vi "LINX - PmodACL2.vi"() -> ()   [LabVIEW 2011]
doc: "PmodACL2\n\nThis example demonstrates how to read 3-axis acceleration values and temperature. \n\nInstructions:\n1. Select the COM Port associated with the LINX device\n2. Select the SPI Channel that the Pmod is connected to.\n3. Select the CS Channel that the Pmod is connected to.\n4. Use the controls to select resolution and data rate\n5. Click the Run Arrow."
uses:
  vi.lib/MakerHub/LINX/Public/Utilities/Open Serial.vi
  vi.lib/MakerHub/LINX/LMH-LINX.lvlib
  vi.lib/MakerHub/LINX/Public/Sensors/Pmods/ACL2/PmodACL2.lvlib
panel:
  out "Loop Rate (Hz)":u32
  out "Waveform Chart":T1(graph)
  in  "Stop Button":bool
  out "Temperature":dbl format="%#_3g"
  in  "Output Data Rate (Hz)":enum16{"400", "200", "100", "50", "25", "12.5"}(ring)=enum."100"
  in  "SPI Channel (0)":u8
  in  "Resolution (g)":enum16{"8g", "4g", "2g"}(ring)=enum."2g"
  in  "CS Channel":u8=10
  in  "Serial Port":refnum<visa-resource-name>="N/A"
  # "PmodACL2\n\nThis example demonstrates how to read 3-axis acceleration values and temperature from PmodACL2. \n\nInstructions:\n1. Select the COM Port associated with the LINX device\n2. Select the SPI Channel that the Pmod is connected to.\n3. Select the CS Channel that the Pmod is connected to.\n4. Use the controls to select resolution and data rate\n5. Click the Run Arrow."
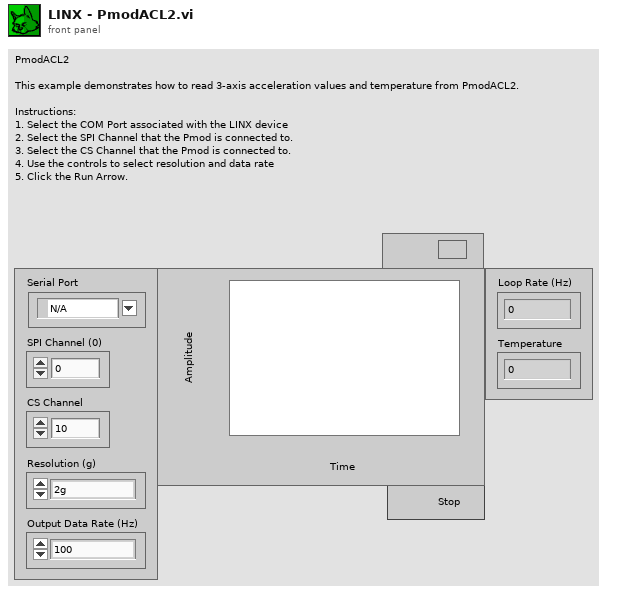
[diagram p1: front panel]
types:
  T1 = cluster{"Numeric Control":dbl, "Numeric Control":dbl, "Numeric Control":dbl}
  T2 = typedef "LMH-LINX.lvlib/LINX Ref.ctl" = cluster{"IO":T3, "Interface":T4, "LINX Device Config":T5}
  T3 = typedef "LMH-LINX.lvlib/Platform.ctl" = enum16{"Remote", "Local"}
  T4 = typedef "LMH-LINX.lvlib/Interface.ctl" = enum16{"Serial", "TCP"}
  T5 = typedef "LMH-LINX.lvlib/Device.lvlib/LINX Device Config.ctl" = cluster{"Interface":T4, "COM Port":refnum<visa-resource-name>, "TCP Configuration":T6, "Device Family":u8, "Device ID":u8, "Device Name":string, "TCP Ref":refnum<k5>, "Channels":T7}
  T6 = typedef "LMH-LINX.lvlib/Device.lvlib/TCP Config.ctl" = cluster{"IP Address":string, "Port":u16}
  T7 = typedef "LMH-LINX.lvlib/Channels.ctl" = cluster{"DI":u8[], "DO":u8[], "AI":u8[], "AO":u8[], "PWM":u8[], "QE":u8[], "UART":u8[], "I2C 2":u8[], "SPI":u8[], "CAN":u8[], "Servo":u8[], "AI Ref (V)":dbl, "AI Resolution (Bits)":u8, "AO Ref (V)":dbl, "AO Resolution (Bits)":u8}
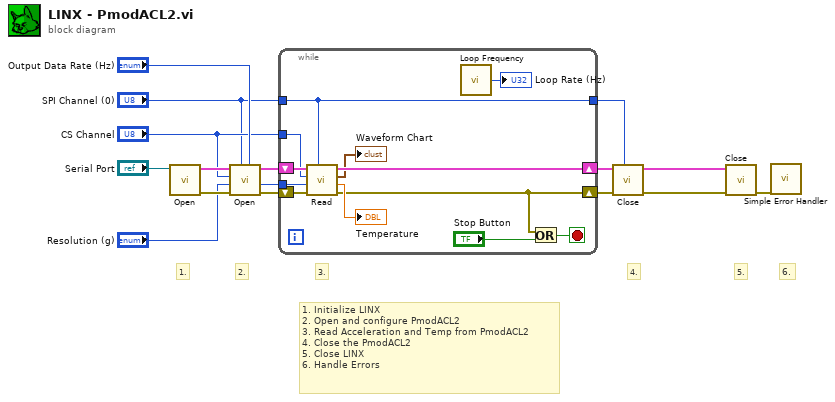
[diagram p0: block diagram]
diagram:
  # "6."
  # "5."
  # "1. Initialize LINX\n2. Open and configure PmodACL2\n3. Read Acceleration and Temp from PmodACL2\n4. Close the PmodACL2\n5. Close LINX\n6. Handle Errors"
  # "4."
  # "3."
  # "2."
  # "1."
  n1 = call-poly "Open.vi"("Serial Port"="Serial Port") -> ("Error Out"=w15:errorcluster, "LINX Resource"=w16:T2)  [unwired: 8 in, 1 out]
  n2 = call "Open.vi"("Output Data Rate (Hz)"="Output Data Rate (Hz)", "SPI Channel (0)"="SPI Channel (0)", "Error In (no error)"=w15, "Resolution (g)"="Resolution (g)", "CS Channel"="CS Channel", "LINX Resource"=w16) -> ("Error Out"=w10:errorcluster, "Resolution (g)"=w9:enum16{"8g", "4g", "2g"}, "LINX Resource"=w11:T2)  [unwired: 3 in]
  n3 = while {
    tunnel: w9 -> [w26]
    tunnel: "CS Channel" -> [w25]
    tunnel: "SPI Channel (0)" -> [w17]
    shift-right: [w24] -> w5
    shift-left: w11 -> [w28]
    shift-right: [w21] -> w6
    shift-left: w10 -> [w27]
    tunnel: [w17] -> w2
    stop <- w22 stop-if-true
    n4 = call "Read.vi"("SPI Channel (0)"=w17, "Error In (no error)"=w27, "Resolution (g)"=w26, "CS Channel"=w25, "LINX Resource"=w28) -> ("Error Out"=w21:errorcluster, "Temperature"=→"Temperature":dbl, "Acceleration Data (g)"=→"Waveform Chart":T1, "LINX Resource"=w24:T2)  [unwired: 3 in]
    n5 = call "Loop Frequency.vi"() -> ("Loop Rate (Hz)"=→"Loop Rate (Hz)":u32)
    n6 = Or(x=w21, y="Stop Button") -> (x .or. y?=w22:bool)
  }
  n7 = call "Close.vi"("SPI Channel (0)"=w2, "Error In"=w6, "LINX Resource"=w5) -> ("Error Out"=w3:errorcluster, "LINX Resource"=w4:T2)  [unwired: 7 in]
  n8 = call "Close.vi"("Error In"=w3, "LINX Resource"=w4) -> ("Error Out"=w1:errorcluster)  [unwired: 9 in]
  n9 = call <vilib>:"Simple Error Handler.vi"("error in (no error)"=w1) -> ()  [unwired: 4 in, 5 out]
